vi "Initialize.vi"(8 "error in (no error)":errorcluster, 11 "Simulated uC in":refnum<class "Simulated uC.lvclass">) -> (0 "error out":errorcluster, 3 "Simulated uC out":refnum<class "Simulated uC.lvclass">)   [LabVIEW 2019, in "Simulated uC.lvclass"]
uses:
  Simulated uC.lvclass
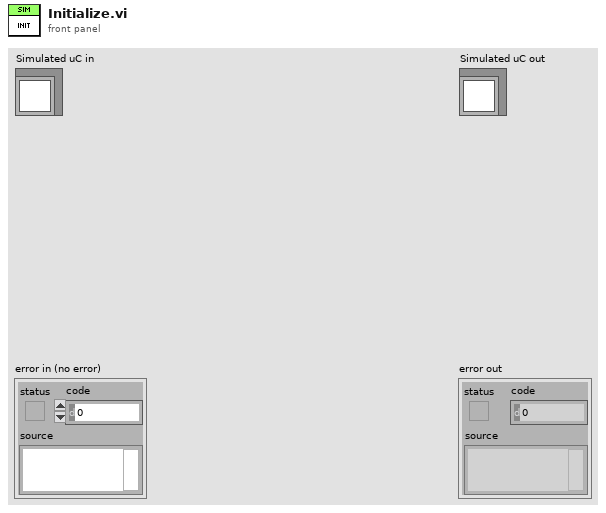
[diagram p1: front panel]
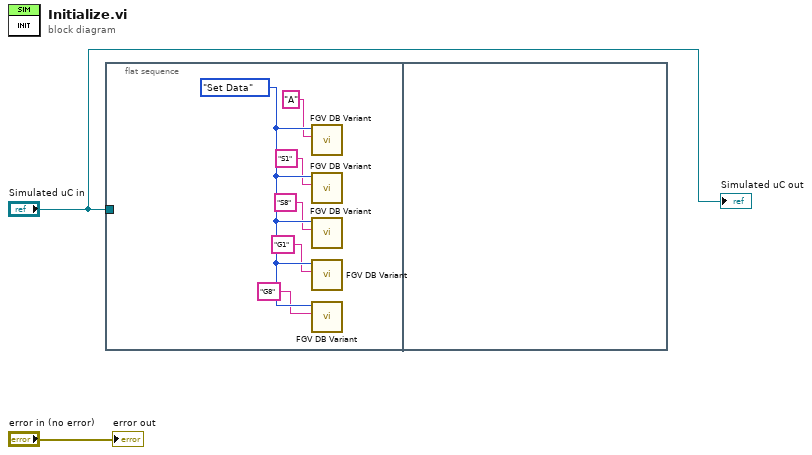
[diagram p0: block diagram]
diagram:
  n1 = flat-sequence {
    tunnel: "Simulated uC in" -> [_]
    frame #0 {
      w8 = enum16{"Set Data", "Get Data", "Reset Data"}."Set Data" ("Opcion")
      n2 = call "FGV DB Variant.vi"("name"="A", "Opcion"=w8) -> ()  [unwired: 7 in, 3 out]
      n3 = call "FGV DB Variant.vi"("name"="S1", "Opcion"=w8) -> ()  [unwired: 7 in, 3 out]
      n4 = call "FGV DB Variant.vi"("name"="S8", "Opcion"=w8) -> ()  [unwired: 7 in, 3 out]
      n5 = call "FGV DB Variant.vi"("name"="G1", "Opcion"=w8) -> ()  [unwired: 7 in, 3 out]
      n6 = call "FGV DB Variant.vi"("name"="G8", "Opcion"=w8) -> ()  [unwired: 7 in, 3 out]
    }
    frame #1 {
    }
  }
  "error out" <- "error in (no error)"
  "Simulated uC out" <- "Simulated uC in"
